vi "laneleftright4.vi"() -> (2 "Coeff right":dbl[](array[numeric]), 3 "Coeff left":dbl[](array[numeric]))   [LabVIEW 2015]
uses:
  G_SEN.vi
  <vilib>/Analysis/1siggen.llb/Ramp Pattern by Delta.vi
  G_LCM.vi
  <vilib>/Analysis/polynomials.llb/1D Polynomial Evaluation (DBL).vi
  G_ALL.vi
  <vilib>/Analysis/NI_AALPro.lvlib
  <vilib>/Analysis/NI_AALBase.lvlib
panel:
  in  "y_gain":dbl min=-1.0 max=1.0
  out "Numeric 2":i32
  out "map_track 2":dbl[][](array[numeric])
  in  "d_safe":dbl=1.0 format="%#_13g"
  out "map_track":dbl[][](array[numeric])
  out "lane_pt":dbl[][](array[numeric])
  in  "x_shift":dbl format="%#_13g"
  in  "y_shift":dbl=-0.0 format="%#_13g"
  in  "x_gain":dbl=0.5 min=-1.0 max=1.0
  out "Lane_C_M":dbl[](array[numeric])=[0.8601491478953653, 0.8717844136967624, 0.882947592858927, 0.8936326403234123, 0.9038337699485205, 0.9135454576426009, 0.9227624443554423, 0.9314797389261423, 0.9396926207859084, 0.9473966425143293, 0.9545876322477319, 0.9612616959383189, 0.9674152194628639, 0.9730448705798238, 0.9781476007338057, 0.9827206467064133, 0.9867615321125792, 0.9902680687415704, 0.993238357741943, 0.9956707906498045, 0.9975640502598242, 0.9989171113385246, 0.9997292411794617, 1.0, 0.9997292411794617, 0.9989171113385246, 0.9975640502598242, 0.9956707906498045, 0.993238357741943, 0.9902680687415704, 0.9867615321125792, 0.9827206467064133]
  out "ratio(-1:left1:right)":dbl
  out "NaN/Path/Refnum?":bool
  out "Rleft":dbl
  out "Rright":dbl
  in  "poly":i32=2 min=1 max=4 step=1
  out "Coeff stop":dbl[](array[numeric])
  out "y_end":dbl[](array[numeric])=[0.8601491478953653, 0.8717844136967624, 0.882947592858927, 0.8936326403234123, 0.9038337699485205, 0.9135454576426009, 0.9227624443554423, 0.9314797389261423, 0.9396926207859084, 0.9473966425143293, 0.9545876322477319, 0.9612616959383189, 0.9674152194628639, 0.9730448705798238, 0.9781476007338057, 0.9827206467064133, 0.9867615321125792, 0.9902680687415704, 0.993238357741943, 0.9956707906498045, 0.9975640502598242, 0.9989171113385246, 0.9997292411794617, 1.0, 0.9997292411794617, 0.9989171113385246, 0.9975640502598242, 0.9956707906498045, 0.993238357741943, 0.9902680687415704, 0.9867615321125792, 0.9827206467064133]
  in  "iter":i32=7
  out "Waveform Graph":dbl[](graph)
  out "w":dbl[](array[numeric])
  out "XY Graph 4":cluster{"Y":dbl[], "Y":dbl[]}[](graph)=[{"Y"=array[3210 elements], "Y"=array[3210 elements]}, {"Y"=[-0.0, 0.001154394197769193, 0.004617650635850623, 0.010389990872226917, 0.018471784248973222, 0.02886354801042046, 0.041565947468740205, 0.056579796217107514, 0.0739060563904701, 0.0935458389742223, 0.11550040416098284, 0.13977116175580306, 0.16635967162997645, 0.19526764422393228, 0.2264969410994837, 0.26004957554195585, 0.2959277132125635, 0.3341336728515216, 0.374669927032528, 0.417539102969144, 0.4627439833735707, 0.5102875073687159, 0.560172771454063, 0.6124030305261954, 0.6669816989546717, 0.7239123517142048, 0.7831987255740245, 0.8448447203451934, 0.9088544001870815, 0.975231994973953, 1.0439819017227023, 1.1151086860829622, 1.1886170838907617, 1.2645120027869723, 1.342798523901962, 1.42348190360768, 1.5065675753387922, 1.592061151484188, 1.6799684253507792, 1.770295373200753, 1.8630481563645134, 1.9582331234307588, 2.0558568125157564, 2.1559259536137603, 2.258447471030621], "Y"=[0.0, 0.5, 1.0, 1.5, 2.0, 2.5, 3.0, 3.5, 4.0, 4.5, 5.0, 5.5, 6.0, 6.5, 7.0, 7.5, 8.0, 8.5, 9.0, 9.5, 10.0, 10.5, 11.0, 11.5, 12.0, 12.5, 13.0, 13.5, 14.0, 14.5, 15.0, 15.5, 16.0, 16.5, 17.0, 17.5, 18.0, 18.5, 19.0, 19.5, 20.0, 20.5, 21.0, 21.5, 22.0]}, {"Y"=[0.362252581831572], "Y"=[-0.8199241909738847]}, {"Y"=array[210 elements], "Y"=array[210 elements]}, {"Y"=[-0.925, -0.925, -0.925, -0.6775, -0.6775, -0.925, -0.925, -0.925, -0.925, -0.6775, -0.6775, -0.925, -0.925, -0.925, 0.9025, 0.9025, 0.9025, 0.6775, 0.6775, 0.9025, 0.9025, 0.9025, 0.9025, 0.6775, 0.6775, 0.9025, 0.9025, 0.9025, -0.925], "Y"=[-0.75, -0.224, 0.224, 0.224, -0.224, -0.224, 0.224, 2.415, 2.885, 2.885, 2.415, 2.415, 2.885, 3.5, 3.5, 2.885, 2.415, 2.415, 2.885, 2.885, 2.415, 0.224, -0.224, -0.224, 0.224, 0.224, -0.224, -0.75, -0.75]}, {"Y"=[0.171875, 0.15377271904051304, 0.1346290179491043, 0.11445423440635205, 0.09325870609283447, 0.07105277068912982, 0.04784676587581635, 0.02365102933347224, -0.0015241012573242174, -0.02766828821599482, -0.05477119386196136, -0.08282248051464558, -0.11181181049346922, -0.14172884611785413, -0.17256324970722198, -0.20430468358099463, -0.23694281005859374, -0.27046729145944115, -0.30486779010295867, -0.340133968308568, -0.3762554883956909, -0.41322201268374914, -0.4510232034921646, -0.4896487231403589], "Y"=[0.0, 0.5, 1.0, 1.5, 2.0, 2.5, 3.0, 3.5, 4.0, 4.5, 5.0, 5.5, 6.0, 6.5, 7.0, 7.5, 8.0, 8.5, 9.0, 9.5, 10.0, 10.5, 11.0, 11.5]}, {"Y"=[1.796875, 1.778772719040513, 1.7596290179491043, 1.739454234406352, 1.7182587060928345, 1.6960527706891297, 1.6728467658758164, 1.6486510293334722, 1.6234758987426758, 1.5973317117840051, 1.5702288061380387, 1.5421775194853544, 1.513188189506531, 1.483271153882146, 1.452436750292778, 1.4206953164190055, 1.3880571899414063, 1.354532708540559, 1.3201322098970414, 1.284866031691432, 1.248744511604309, 1.2117779873162509, 1.1739767965078354, 1.135351276859641, 1.0959117660522462, 1.0556686017662287, 1.014632121682167, 0.9728126634806396, 0.9302205648422242, 0.8868661634474992], "Y"=[0.0, 0.5, 1.0, 1.5, 2.0, 2.5, 3.0, 3.5, 4.0, 4.5, 5.0, 5.5, 6.0, 6.5, 7.0, 7.5, 8.0, 8.5, 9.0, 9.5, 10.0, 10.5, 11.0, 11.5, 12.0, 12.5, 13.0, 13.5, 14.0, 14.5]}, {"Y"=[-1.453125, -1.471227280959487, -1.4903709820508957, -1.510545765593648, -1.5317412939071655, -1.5539472293108703, -1.5771532341241836, -1.6013489706665278, -1.6265241012573242, -1.6526682882159949, -1.6797711938619613, -1.7078224805146456, -1.736811810493469, -1.766728846117854, -1.797563249707222, -1.8293046835809945, -1.8619428100585937, -1.895467291459441, -1.9298677901029586], "Y"=[0.0, 0.5, 1.0, 1.5, 2.0, 2.5, 3.0, 3.5, 4.0, 4.5, 5.0, 5.5, 6.0, 6.5, 7.0, 7.5, 8.0, 8.5, 9.0]}, {"Y"=[0.171875, 0.2568230007600336, 0.3384052130063493, 0.44574342526006827, 0.5205081969556753, 0.5917680690742042, 0.659409530134929, 0.7229937549325056, 0.7835496148685115, 0.8405449546633443, 0.9258576868463875], "Y"=[-20.239964538708662, -19.725637940364884, -19.211158961966362, -18.6998967366845, -18.19022720070031, -17.681887266143153, -17.17615515566314, -16.67683575591291, -16.176265245349786, -15.679082775270938, -15.183754484614711]}, {"Y"=[7.134647485270904], "Y"=[38.71960961082238]}, {"Y"=array[980 elements], "Y"=array[980 elements]}, {"Y"=[], "Y"=[]}]
  out "y":dbl[](array[numeric])
  out "x":dbl[](array[numeric])
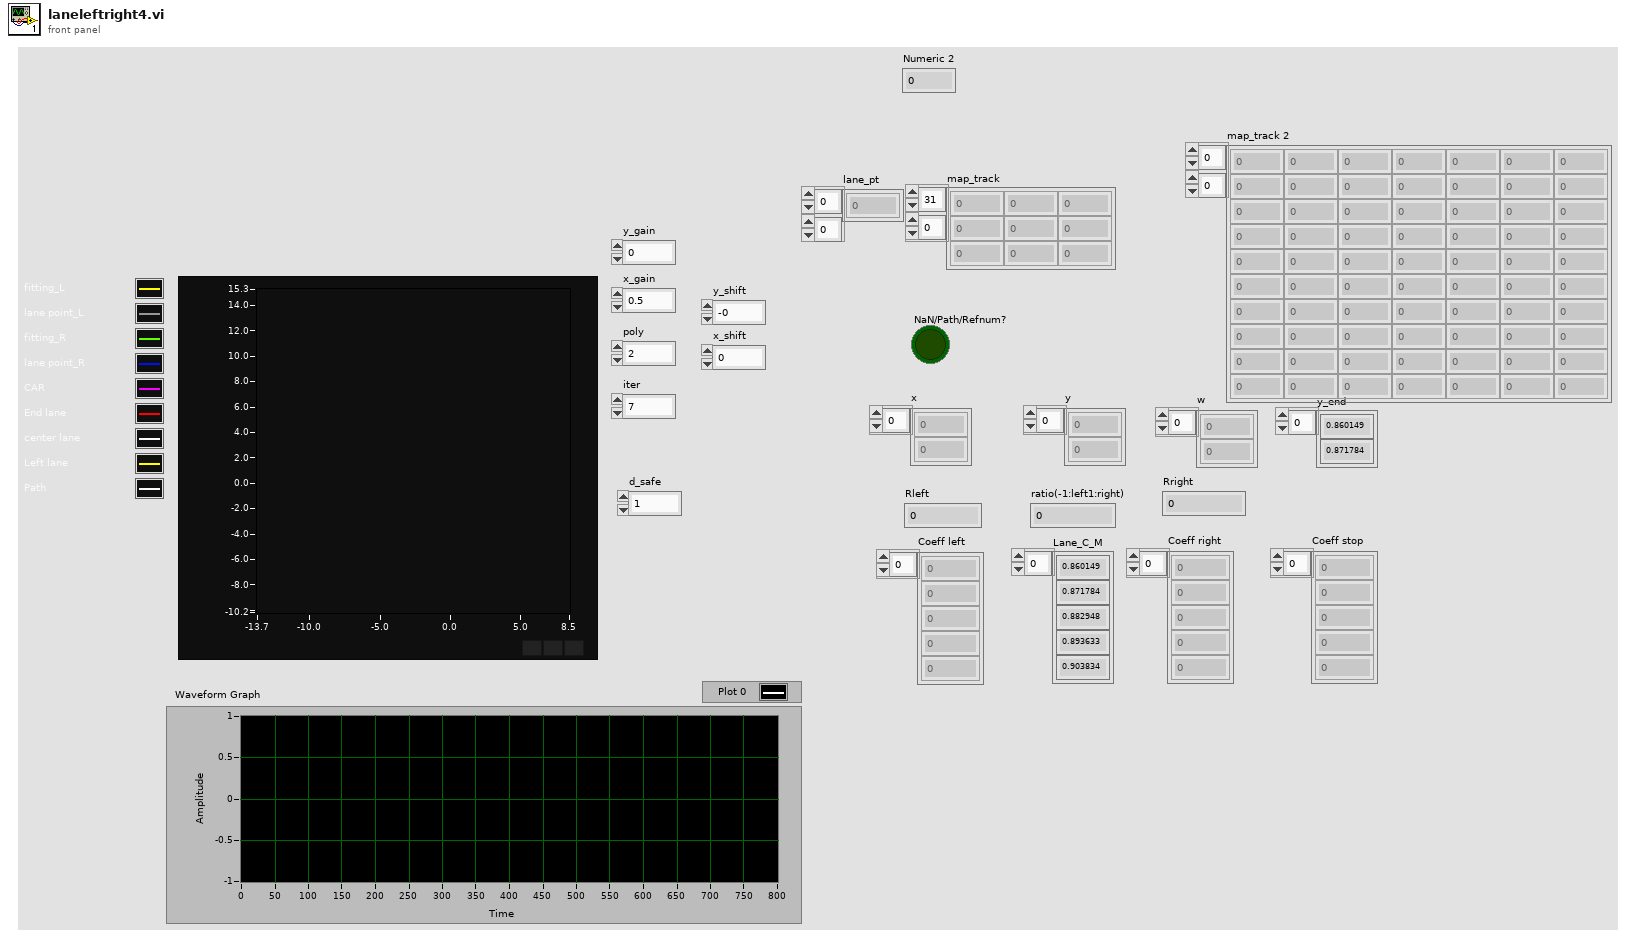
[diagram p1: front panel]
types:
  T1 = cluster{"hash":i64, "sys time":i64, "size":i64, "x":dbl[], "y":dbl[]}
  T2 = cluster{"delta":bool, "Rotational position":dbl, "Rotational position":dbl}[]
  T3 = cluster{"C_Wheel base":dbl, "ratio_steer":dbl, "Overall width":dbl, "af":dbl, "turn radius":dbl, "eval":dbl, "ap":dbl, "an":dbl, "Vmax":dbl, "mu":dbl, "Vlast":dbl}
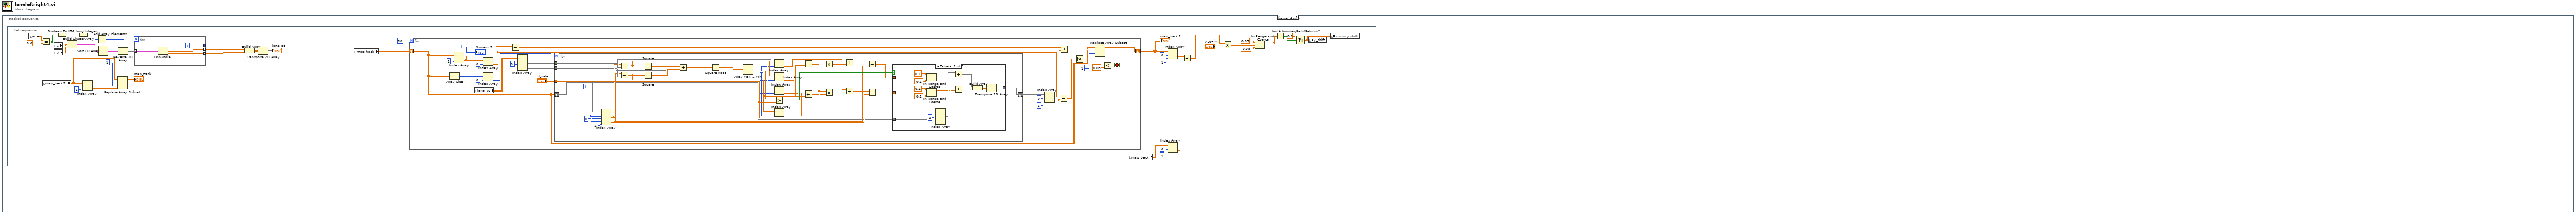
[diagram p0: block diagram]
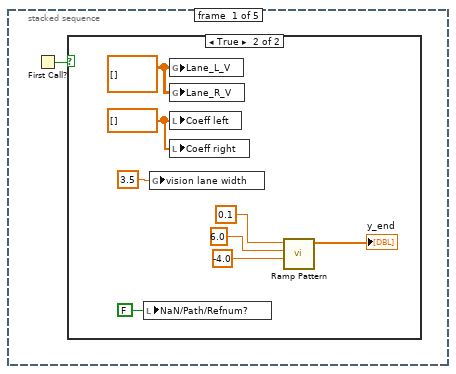
[diagram p2: hidden frame]
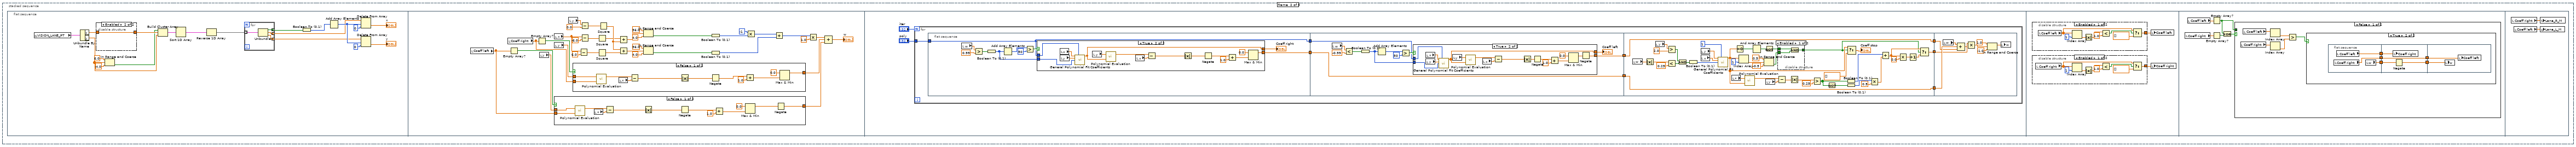
[diagram p4: hidden frame]
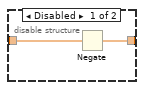
[diagram p5: hidden frame]
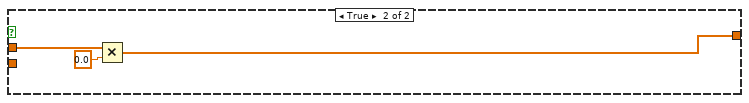
[diagram p6: hidden frame]
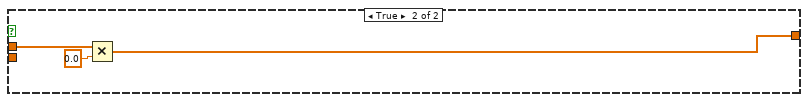
[diagram p7: hidden frame]
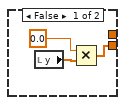
[diagram p8: hidden frame]
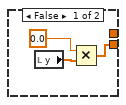
[diagram p9: hidden frame]
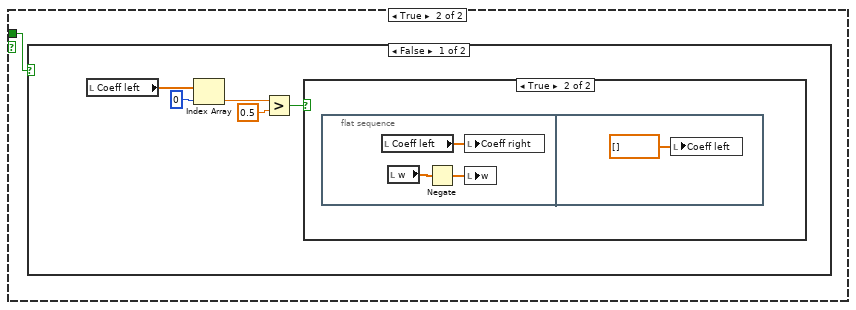
[diagram p14: hidden frame]
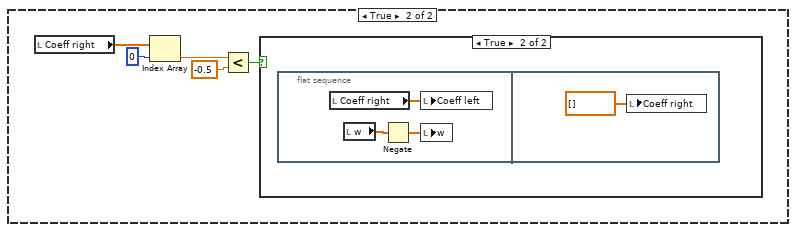
[diagram p16: hidden frame]
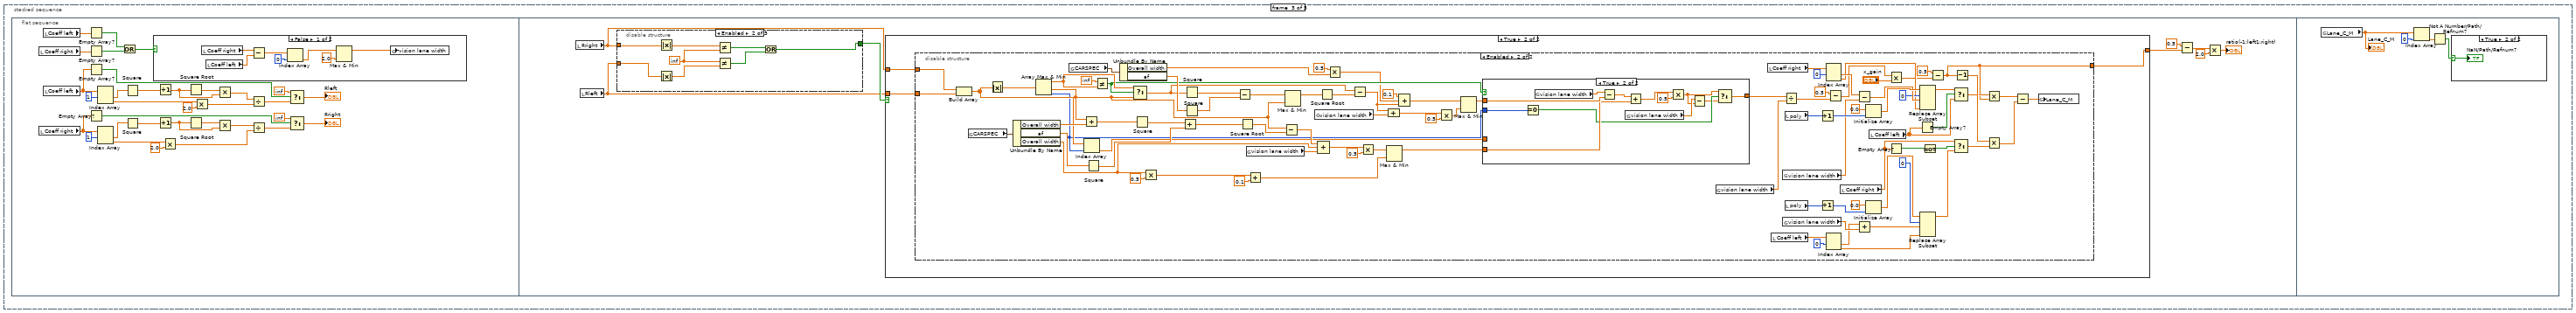
[diagram p18: hidden frame]
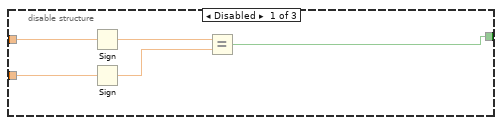
[diagram p20: hidden frame]
diagram:
  n1 = stacked-sequence {
    frame #0 {
      n2 = First Call?() -> (First Call?: T/F=w1:bool)
      n3 = case shown="True" w1 {
        frame False {
        }
        frame True {
          w2 = dbl[] [] ("Coeff left")
          w4 = dbl[][] [] ("Lane_R_V")
          n4 = local write "NaN/Path/Refnum?"(FALSE ("NaN/Path/Refnum?")) -> ()
          n5 = global write "G_SEN.vi" "vision lane width"(3.5 ("vision lane width")) -> ()
          n6 = global write "G_SEN.vi" "Lane_L_V"(w4) -> ()
          n7 = global write "G_SEN.vi" "Lane_R_V"(w4) -> ()
          n8 = local write "Coeff left"(w2) -> ()
          n9 = local write "Coeff right"(w2) -> ()
          n10 = call-poly <vilib>:"Ramp Pattern.vi"("start"=-4.0, "end"=6.0, "delta"=0.1) -> ("Ramp Pattern"=→"y_end":dbl[])  [unwired: 6 in, 2 out]
        }
      }
    }
    frame #1 {
      n11 = flat-sequence {
        frame #0 {
          n12 = global read "G_LCM.vi" "VISION_LANE_PT"() -> (w10:T1)
          n13 = Unbundle By Name(w10) -> ("x"=w27:dbl[], "y"=w21:dbl[])
          n14 = disable-structure shown="Enabled" {
            disable-tunnel: w27 -> [w30 w31]
            disable-tunnel: [w29 w31] -> w28
            frame Disabled {
              n15 = Negate(x=w30) -> (-x=w29:dbl[])
            }
            frame Enabled {
            }
          }
          n16 = In Range and Coerce(upper limit=6.0 ("delta"), x=w21, lower limit=-4.0) -> (In Range?=w19:bool[])  [unwired: 1 out]
          n17 = Build Cluster Array(w19, w28, w21) -> (w17:T2)
          n18 = Sort 1D Array(array=w17) -> (sorted array=w18:T2)
          n19 = Reverse 1D Array(array=w18) -> (reversed array=w12:T2)
          n20 = for {
            tunnel: w12 -> [w35] mode=indexing
            tunnel: [w34] -> w14 mode=indexing
            tunnel: [w33] -> w15 mode=indexing
            tunnel: [w32] -> w22 mode=indexing
            n21 = Unbundle(w35) -> ("delta"=w32:bool, "Rotational position"=w34:dbl, "Rotational position"=w33:dbl)
          }
          n22 = Boolean To (0,1)(Boolean=w22) -> (0, 1=w13:i16[])
          n23 = Add Array Elements(numeric array=w13) -> (sum=w23:i16)
          n24 = Delete From Array(array=w14, length=w23, index=0) -> (deleted portion=→"x":dbl[])  [unwired: 1 out]
          n25 = Delete From Array(array=w15, length=w23, index=0) -> (deleted portion=→"y":dbl[])  [unwired: 1 out]
        }
        frame #1 {
          n26 = local read "Coeff left"() -> (w67:dbl[])
          n27 = local read "Coeff right"() -> (w66:dbl[])
          n28 = Empty Array?(array=w67) -> (empty?=w68:bool)
          n29 = Empty Array?(array=w66) -> (empty?=w69:bool)
          n30 = local read "y"() -> (w64:dbl[])
          n31 = local read "x"() -> (w36:dbl[])
          n32 = local read "y"() -> (w70:dbl[])
          n33 = case shown="False" w68 {
            tunnel: w64 -> [w90 w98]
            tunnel: w67 -> [w87 _]
            tunnel: [w85 w97] -> w65
            frame False {
              n34 = call-poly <vilib>:"Polynomial Evaluation.vi"("P(x)"=w87, "A"=w90) -> ("P(A)"=w89:dbl[])  [unwired: 1 out]
              n35 = local read "x"() -> (w88:dbl[])
              n36 = Subtract(x=w89, y=w88) -> (x-y=w94:dbl[])
              n37 = Absolute Value(x=w94) -> (abs(x)=w93:dbl[])
              n38 = Negate(x=w93) -> (-x=w92:dbl[])
              n39 = Add(x=w92, y=1.0) -> (x+y=w96:dbl[])
              n40 = Max & Min(x=0.0, y=w96) -> (max(x,y)=w86:dbl[])  [unwired: 1 out]
              n41 = Negate(x=w86) -> (-x=w85:dbl[])
            }
            frame True {
              n42 = Multiply(x=w98, y=0.0) -> (x*y=w97:dbl[])
            }
          }
          n43 = local read "y"() -> (w37:dbl[])
          n44 = case shown="False" w69 {
            tunnel: [w79 w82] -> w62
            tunnel: w66 -> [w78 _]
            tunnel: w70 -> [w71 w83]
            frame False {
              n45 = call-poly <vilib>:"Polynomial Evaluation.vi"("P(x)"=w78, "A"=w71) -> ("P(A)"=w76:dbl[])  [unwired: 1 out]
              n46 = local read "x"() -> (w77:dbl[])
              n47 = Subtract(x=w76, y=w77) -> (x-y=w72:dbl[])
              n48 = Absolute Value(x=w72) -> (abs(x)=w73:dbl[])
              n49 = Negate(x=w73) -> (-x=w74:dbl[])
              n50 = Add(x=w74, y=1.0) -> (x+y=w80:dbl[])
              n51 = Max & Min(x=0.0, y=w80) -> (max(x,y)=w79:dbl[])  [unwired: 1 out]
            }
            frame True {
              n52 = Multiply(x=w83, y=0.0) -> (x*y=w82:dbl[])
            }
          }
          n53 = Subtract(x=w36, y=6.0) -> (x-y=w40:dbl[])
          n54 = Subtract(x=w37, y=0.0) -> (x-y=w49:dbl[])
          n55 = Subtract(x=w36, y=-6.0) -> (x-y=w42:dbl[])
          n56 = Square(x=w42) -> (x^2=w41:dbl[])
          n57 = Square(x=w40) -> (x^2=w50:dbl[])
          n58 = Square(x=w49) -> (x^2=w51:dbl[])
          n59 = Add(x=w41, y=w51) -> (x+y=w57:dbl[])
          n60 = Add(x=w51, y=w50) -> (x+y=w52:dbl[])
          n61 = In Range and Coerce(upper limit=36.0, x=w57, lower limit=4.0) -> (In Range?=w59:bool[])  [unwired: 1 out]
          n62 = In Range and Coerce(upper limit=36.0, x=w52, lower limit=4.0) -> (In Range?=w58:bool[])  [unwired: 1 out]
          n63 = Boolean To (0,1)(Boolean=w59) -> (0, 1=w60:i16[])
          n64 = Boolean To (0,1)(Boolean=w58) -> (0, 1=w61:i16[])
          n65 = Multiply(x=i16 -1, y=w60) -> (x*y=w45:i16[])
          n66 = Add(x=w45, y=w61) -> (x+y=w47:i16[])
          n67 = Multiply(x=w47, y=1.0 ("element")) -> (x*y=w63:dbl[])
          n68 = Compound Arithmetic op=ADD(w63, w62, w65) -> (→"w":dbl[])
        }
        frame #2 {
          n69 = for {
            N: "iter" -> [_]
            tunnel: "poly" -> [w103]
            n70 = flat-sequence {
              tunnel: [w117] -> w109
              tunnel: w103 -> [w110]
              tunnel: [w110] -> w102
              tunnel: [w148] -> w108
              tunnel: w109 -> [w148]
              tunnel: [w145] -> w106
              tunnel: w102 -> [w138]
              tunnel: w108 -> [w210]
              tunnel: [w210] -> w107
              tunnel: w106 -> [w209]
              tunnel: [w209] -> w105
              tunnel: [w180] -> w104
              tunnel: w107 -> [w218]
              tunnel: w105 -> [w217]
              tunnel: w104 -> [w216]
              frame #0 {
                n71 = local read "w"() -> (w119:dbl[])
                n72 = Greater?(x=w119, y=0.99) -> (0:w111:bool[])
                n73 = Boolean To (0,1)(Boolean=w111) -> (0, 1=w112:i16[])
                n74 = Add Array Elements(numeric array=w112) -> (sum=w115:i16)
                n75 = Greater?(x=w115, y=i16 50) -> (0:w113:bool)
                n76 = case shown="True" w113 {
                  tunnel: [w121 w128] -> w117
                  tunnel: [_ w127] -> w116
                  tunnel: w112 -> [_ w124]
                  tunnel: w110 -> [_ w123]
                  frame False {
                    n77 = local read "y"() -> (w122:dbl[])
                    n78 = Multiply(x=0.0, y=w122) -> (x*y=w121:dbl[])
                  }
                  frame True {
                    n79 = local read "x"() -> (w125:dbl[])
                    n80 = local read "y"() -> (w126:dbl[])
                    n81 = call <vilib>:"General Polynomial Fit Coefficients.vi"("Y"=w125, "polynomial order"=w123, "X"=w126, "Weight"=w124) -> ("Polynomial Coefficients"=w127:dbl[])  [unwired: 10 in, 1 out]
                    n82 = local read "y"() -> (w137:dbl[])
                    n83 = call-poly <vilib>:"Polynomial Evaluation.vi"("P(x)"=w127, "A"=w137) -> ("P(A)"=w136:dbl[])  [unwired: 1 out]
                    n84 = local read "x"() -> (w135:dbl[])
                    n85 = Subtract(x=w136, y=w135) -> (x-y=w134:dbl[])
                    n86 = Absolute Value(x=w134) -> (abs(x)=w133:dbl[])
                    n87 = Negate(x=w133) -> (-x=w132:dbl[])
                    n88 = Add(x=w132, y=1.0) -> (x+y=w129:dbl[])
                    n89 = Max & Min(x=0.0, y=w129) -> (max(x,y)=w128:dbl[])  [unwired: 1 out]
                  }
                }
                "Coeff right" <- w116
              }
              frame #1 {
                n90 = local read "w"() -> (w146:dbl[])
                n91 = Less?(x=w146, y=-0.99) -> (x < y?=w141:bool[])
                n92 = Boolean To (0,1)(Boolean=w141) -> (0, 1=w139:i16[])
                n93 = Add Array Elements(numeric array=w139) -> (sum=w142:i16)
                n94 = Greater?(x=w142, y=i16 50) -> (0:w140:bool)
                n95 = case shown="True" w140 {
                  tunnel: [w149 w157] -> w145
                  tunnel: [_ w156] -> w144
                  tunnel: w139 -> [_ w153]
                  tunnel: w138 -> [_ w152]
                  frame False {
                    n96 = local read "y"() -> (w150:dbl[])
                    n97 = Multiply(x=0.0, y=w150) -> (x*y=w149:dbl[])
                  }
                  frame True {
                    n98 = local read "x"() -> (w154:dbl[])
                    n99 = local read "y"() -> (w155:dbl[])
                    n100 = call <vilib>:"General Polynomial Fit Coefficients.vi"("Y"=w154, "polynomial order"=w152, "X"=w155, "Weight"=w153) -> ("Polynomial Coefficients"=w156:dbl[])  [unwired: 10 in, 1 out]
                    n101 = local read "y"() -> (w161:dbl[])
                    n102 = call-poly <vilib>:"Polynomial Evaluation.vi"("P(x)"=w156, "A"=w161) -> ("P(A)"=w162:dbl[])  [unwired: 1 out]
                    n103 = local read "x"() -> (w163:dbl[])
                    n104 = Subtract(x=w162, y=w163) -> (x-y=w164:dbl[])
                    n105 = Absolute Value(x=w164) -> (abs(x)=w165:dbl[])
                    n106 = Negate(x=w165) -> (-x=w159:dbl[])
                    n107 = Add(x=w159, y=1.0) -> (x+y=w166:dbl[])
                    n108 = Max & Min(x=0.0, y=w166) -> (max(x,y)=w160:dbl[])  [unwired: 1 out]
                    n109 = Negate(x=w160) -> (-x=w157:dbl[])
                  }
                }
                "Coeff left" <- w144
              }
              frame #2 {
                n110 = local read "w"() -> (w188:dbl[])
                n111 = Absolute Value(x=w188) -> (abs(x)=w187:dbl[])
                n112 = local read "y"() -> (w192:dbl[])
                n113 = Greater?(x=w192, y=2.0) -> (0:w190:bool[])
                n114 = Less?(x=w187, y=0.25) -> (x < y?=w186:bool[])
                n115 = And(x=w190, y=w186) -> (x .and. y?=w189:bool[])
                n116 = Boolean To (0,1)(Boolean=w189) -> (0, 1=w208:i16[])
                n117 = local read "y"() -> (w202:dbl[])
                n118 = local read "x"() -> (w201:dbl[])
                n119 = call <vilib>:"General Polynomial Fit Coefficients.vi"("Y"=w202, "polynomial order"=1, "X"=w201, "Weight"=w208) -> ("Polynomial Coefficients"=w173:dbl[])  [unwired: 10 in, 1 out]
                n120 = local read "x"() -> (w206:dbl[])
                n121 = Equal To 0?(x=w173) -> (x = 0?=w172:bool[])
                n122 = Index Array(array=w173, index=1) -> (element=w183:dbl)
                n123 = call-poly <vilib>:"Polynomial Evaluation.vi"("P(x)"=w173, "A"=w206) -> ("P(A)"=w205:dbl[])  [unwired: 1 out]
                n124 = And Array Elements(Boolean array=w172) -> (logical AND=w169:bool)
                n125 = In Range and Coerce(upper limit=0.5, x=w183, lower limit=-0.5) -> (In Range?=w171:bool)  [unwired: 1 out]
                n126 = Not(x=w169) -> (.not. x?=w168:bool)
                n127 = local read "y"() -> (w204:dbl[])
                n128 = Subtract(x=w205, y=w204) -> (x-y=w203:dbl[])
                n129 = disable-structure shown="Enabled" {
                  disable-tunnel: w171 -> [w213 _]
                  disable-tunnel: [w212 _] -> w170
                  disable-tunnel: w168 -> [w211 _]
                  frame Enabled {
                    n130 = And(x=w211, y=w213) -> (x .and. y?=w212:bool)
                  }
                  frame Disabled {
                  }
                }
                n131 = Absolute Value(x=w203) -> (abs(x)=w200:dbl[])
                n132 = Greater?(x=w200, y=0.25 ("Numeric 2")) -> (0:w198:bool[])
                n133 = Not(x=w198) -> (.not. x?=w197:bool[])
                n134 = Boolean To (0,1)(Boolean=w198) -> (0, 1=w193:i16[])
                n135 = Boolean To (0,1)(Boolean=w197) -> (0, 1=w196:i16[])
                n136 = Select(t=w173, s=w170, f=dbl[] []) -> (s? t:f=→"Coeff stop":dbl[])
                n137 = Multiply(x=w196, y=0.5) -> (x*y=w194:dbl[])
                n138 = Add(x=w193, y=w194) -> (x+y=w179:dbl[])
                n139 = Multiply(x=w179, y=0.0) -> (x*y=w177:dbl[])
                n140 = Increment(x=w177) -> (x+1=w176:dbl[])
                n141 = Select(t=w179, s=w170, f=w176) -> (s? t:f=w180:dbl[])
              }
              frame #3 {
                n142 = local read "w"() -> (w222:dbl[])
                n143 = Compound Arithmetic op=ADD(w222, w218, w217) -> (w215:dbl[])
                n144 = Multiply(x=w216, y=w215) -> (x*y=w214:dbl[])
                n145 = In Range and Coerce(upper limit=1.0, x=w214, lower limit=-1.0) -> (coerced(x)=w219:dbl[])  [unwired: 1 out]
                n146 = local write "w"(w219) -> ()
              }
            }
          }
        }
        frame #3 {
          n147 = disable-structure shown="Enabled" {
            disable-tunnel: [w226 _] -> w223
            frame Enabled {
              n148 = local read "Coeff left"() -> (w225:dbl[])
              n149 = Index Array(array=w225, index=1) -> (element=w228:dbl)
              n150 = Absolute Value(x=w228) -> (abs(x)=w229:dbl)
              n151 = Less?(x=w229, y=1.0) -> (x < y?=w231:bool)
              n152 = Select(t=w225, s=w231, f=dbl[] []) -> (s? t:f=w226:dbl[])
            }
            frame Disabled {
            }
          }
          n153 = disable-structure shown="Enabled" {
            disable-tunnel: [w235 _] -> w224
            frame Enabled {
              n154 = local read "Coeff right"() -> (w233:dbl[])
              n155 = Index Array(array=w233, index=1) -> (element=w239:dbl)
              n156 = Absolute Value(x=w239) -> (abs(x)=w238:dbl)
              n157 = Less?(x=w238, y=1.0) -> (x < y?=w236:bool)
              n158 = Select(t=w233, s=w236, f=dbl[] []) -> (s? t:f=w235:dbl[])
            }
            frame Disabled {
            }
          }
          n159 = local write "Coeff left"(w223) -> ()
          n160 = local write "Coeff right"(w224) -> ()
        }
        frame #4 {
          n161 = local read "Coeff right"() -> (w242:dbl[])
          n162 = local read "Coeff left"() -> (w241:dbl[])
          n163 = Empty Array?(array=w241) -> (empty?=w245:bool)
          n164 = Empty Array?(array=w242) -> (empty?=w243:bool)
          n165 = Exclusive Or(1:w243, 2:w245) -> (0:w244:bool)
          n166 = case shown="False" w244 {
            tunnel: w245 -> [_ w265]
            frame False {
              n167 = local read "Coeff right"() -> (w249:dbl[])
              n168 = local read "Coeff left"() -> (w250:dbl[])
              n169 = Index Array(array=w250) -> (element=w248:dbl)  [unwired: 1 in]
              n170 = Index Array(array=w249) -> (element=w247:dbl)  [unwired: 1 in]
              n171 = Greater?(x=w248, y=w247) -> (0:w246:bool)
              n172 = case shown="True" w246 {
                frame False {
                }
                frame True {
                  n173 = flat-sequence {
                    tunnel: [w258] -> w254
                    tunnel: [w257] -> w253
                    tunnel: [w256] -> w252
                    tunnel: [w262] -> w255
                    tunnel: w254 -> [w262]
                    tunnel: w253 -> [w261]
                    tunnel: w252 -> [w260]
                    tunnel: [w259] -> w251
                    tunnel: w255 -> [w264]
                    tunnel: w251 -> [w263]
                    frame #0 {
                      n174 = local read "Coeff right"() -> (w258:dbl[])
                      n175 = local read "Coeff left"() -> (w257:dbl[])
                      n176 = local read "w"() -> (w256:dbl[])
                    }
                    frame #1 {
                      n177 = local write "Coeff right"(w261) -> ()
                      n178 = Negate(x=w260) -> (-x=w259:dbl[])
                    }
                    frame #2 {
                      n179 = local write "w"(w263) -> ()
                      n180 = local write "Coeff left"(w264) -> ()
                    }
                  }
                }
              }
            }
            frame True {
              n181 = case shown="False" w265 {
                frame False {
                  n182 = local read "Coeff left"() -> (w270:dbl[])
                  n183 = Index Array(array=w270, index=0) -> (element=w268:dbl)
                  n184 = Greater?(x=w268, y=0.5) -> (0:w266:bool)
                  n185 = case shown="True" w266 {
                    frame False {
                    }
                    frame True {
                      n186 = flat-sequence {
                        frame #0 {
                          n187 = local read "Coeff left"() -> (w273:dbl[])
                          n188 = local read "w"() -> (w272:dbl[])
                          n189 = Negate(x=w272) -> (-x=w271:dbl[])
                          n190 = local write "Coeff right"(w273) -> ()
                          n191 = local write "w"(w271) -> ()
                        }
                        frame #1 {
                          n192 = local write "Coeff left"(dbl[] []) -> ()
                        }
                      }
                    }
                  }
                }
                frame True {
                  n193 = local read "Coeff right"() -> (w279:dbl[])
                  n194 = Index Array(array=w279, index=0) -> (element=w277:dbl)
                  n195 = Less?(x=w277, y=-0.5) -> (x < y?=w275:bool)
                  n196 = case shown="True" w275 {
                    frame False {
                    }
                    frame True {
                      n197 = flat-sequence {
                        frame #0 {
                          n198 = local read "Coeff right"() -> (w282:dbl[])
                          n199 = local read "w"() -> (w281:dbl[])
                          n200 = Negate(x=w281) -> (-x=w280:dbl[])
                          n201 = local write "Coeff left"(w282) -> ()
                          n202 = local write "w"(w280) -> ()
                        }
                        frame #1 {
                          n203 = local write "Coeff right"(dbl[] []) -> ()
                        }
                      }
                    }
                  }
                }
              }
            }
          }
        }
        frame #5 {
          n204 = local read "Coeff right"() -> (w285:dbl[])
          n205 = local read "Coeff left"() -> (w284:dbl[])
          n206 = global write "G_SEN.vi" "Lane_R_M"(w285) -> ()
          n207 = global write "G_SEN.vi" "Lane_L_M"(w284) -> ()
        }
      }
    }
    frame #2 {
      n208 = flat-sequence {
        frame #0 {
          n209 = local read "Coeff right"() -> (w287:dbl[])
          n210 = local read "Coeff right"() -> (w315:dbl[])
          n211 = local read "Coeff left"() -> (w286:dbl[])
          n212 = local read "Coeff left"() -> (w313:dbl[])
          n213 = Empty Array?(array=w286) -> (empty?=w289:bool)
          n214 = Empty Array?(array=w287) -> (empty?=w290:bool)
          n215 = Empty Array?(array=w313) -> (empty?=w307:bool)
          n216 = Empty Array?(array=w315) -> (empty?=w309:bool)
          n217 = Index Array(array=w313, index #1=1 ("index")) -> (element #1=w306:dbl, element #2=w299:dbl)  [unwired: 1 in]
          n218 = Index Array(array=w315, index #1=1 ("index")) -> (element #1=w291:dbl, element #2=w298:dbl)  [unwired: 1 in]
          n219 = Or(x=w289, y=w290) -> (x .or. y?=w288:bool)
          n220 = Square(x=w306) -> (x^2=w305:dbl)
          n221 = Square(x=w291) -> (x^2=w292:dbl)
          n222 = case shown="False" w288 {
            frame False {
              n223 = local read "Coeff right"() -> (w322:dbl[])
              n224 = local read "Coeff left"() -> (w319:dbl[])
              n225 = Subtract(x=w322, y=w319) -> (x-y=w320:dbl[])
              n226 = Index Array(array=w320, index=0) -> (element=w323:dbl)
              n227 = Max & Min(x=w323, y=2.0) -> (max(x,y)=w324:dbl)  [unwired: 1 out]
              n228 = global write "G_SEN.vi" "vision lane width"(w324) -> ()
            }
            frame True {
            }
          }
          n229 = Increment(x=w305) -> (x+1=w303:dbl)
          n230 = Increment(x=w292) -> (x+1=w294:dbl)
          n231 = Multiply(x=w298, y=2.0) -> (x*y=w296:dbl)
          n232 = Square Root(x=w303) -> (sqrt(x)=w304:dbl)
          n233 = Square Root(x=w294) -> (sqrt(x)=w293:dbl)
          n234 = Multiply(x=w299, y=2.0) -> (x*y=w301:dbl)
          n235 = Multiply(x=w304, y=w303) -> (x*y=w302:dbl)
          n236 = Multiply(x=w293, y=w294) -> (x*y=w295:dbl)
          n237 = Divide(x=w302, y=w301) -> (x/y=w308:dbl)
          n238 = Divide(x=w295, y=w296) -> (x/y=w310:dbl)
          n239 = Select(t=inf, s=w307, f=w308) -> (s? t:f=→"Rleft":dbl)
          n240 = Select(t=inf, s=w309, f=w310) -> (s? t:f=→"Rright":dbl)
        }
        frame #1 {
          n241 = local read "Rright"() -> (w326:dbl)
          n242 = local read "Rleft"() -> (w327:dbl)
          n243 = disable-structure shown="Enabled" {
            disable-tunnel: w326 -> [w338 w345 _]
            disable-tunnel: w327 -> [w337 w346 _]
            disable-tunnel: [w334 w341 TRUE] -> w328
            frame Disabled {
              n244 = Sign(1:w338) -> (0:w336:dbl)
              n245 = Sign(1:w337) -> (0:w335:dbl)
              n246 = Equal?(x=w336, y=w335) -> (x = y?=w334:bool)
            }
            frame Enabled {
              w343 = inf
              n247 = Absolute Value(x=w345) -> (abs(x)=w344:dbl)
              n248 = Absolute Value(x=w346) -> (abs(x)=w342:dbl)
              n249 = Not Equal?(x=w344, y=w343) -> (x != y?=w340:bool)
              n250 = Not Equal?(x=w343, y=w342) -> (x != y?=w339:bool)
              n251 = Or(x=w340, y=w339) -> (x .or. y?=w341:bool)
            }
            frame Disabled {
            }
          }
          n252 = case shown="True" w328 {
            tunnel: w326 -> [_ w383]
            tunnel: w327 -> [_ w382]
            tunnel: [0.5 w381] -> w329
            frame False {
              n253 = local read "Coeff right"() -> (w352:dbl[])
              n254 = local read "Coeff left"() -> (w353:dbl[])
              n255 = Empty Array?(array=w352) -> (empty?=w351:bool)
              n256 = Empty Array?(array=w353) -> (empty?=w349:bool)
              n257 = Exclusive Or(1:w351, 2:w349) -> (0:w350:bool)
              n258 = case shown="True" w350 {
                tunnel: w349 -> [w354 w362]
                frame False {
                  n259 = case shown="True" w354 {
                    frame False {
                      w355 = 0.5
                      n260 = local read "Coeff right"() -> (w359:dbl[])
                      n261 = local read "Coeff left"() -> (w361:dbl[])
                      n262 = Decrement(x=w355) -> (x-1=w360:dbl)
                      n263 = Multiply(x=w361, y=w355) -> (x*y=w358:dbl[])
                      n264 = Multiply(x=w360, y=w359) -> (x*y=w357:dbl[])
                      n265 = Subtract(x=w358, y=w357) -> (x-y=w356:dbl[])
                      n266 = global write "G_SEN.vi" "Lane_C_M"(w356) -> ()
                    }
                    frame True {
                    }
                  }
                }
                frame True {
                  n267 = case shown="False" w362 {
                    frame False {
                      n268 = global read "G_SEN.vi" "vision lane width"() -> (w365:dbl)
                      n269 = local read "Coeff left"() -> (w371:dbl[])
                      n270 = Index Array(array=w371, index=0) -> (element=w369:dbl)
                      n271 = Multiply(x=w365, y=0.5) -> (x*y=w363:dbl)
                      n272 = Add(x=w369, y=w363) -> (x+y=w368:dbl)
                      n273 = Replace Array Subset(array=w371, new element=w368, index=0) -> (w366:dbl[])
                      n274 = global write "G_SEN.vi" "Lane_C_M"(w366) -> ()
                    }
                    frame True {
                      n275 = global read "G_SEN.vi" "vision lane width"() -> (w374:dbl)
                      n276 = local read "Coeff right"() -> (w380:dbl[])
                      n277 = Index Array(array=w380, index=0) -> (element=w378:dbl)
                      n278 = Multiply(x=w374, y=0.5) -> (x*y=w372:dbl)
                      n279 = Subtract(x=w378, y=w372) -> (x-y=w377:dbl)
                      n280 = Replace Array Subset(array=w380, new element=w377, index=0) -> (w375:dbl[])
                      n281 = global write "G_SEN.vi" "Lane_C_M"(w375) -> ()
                    }
                  }
                }
              }
            }
            frame True {
              n282 = disable-structure shown="Enabled" {
                disable-tunnel: w383 -> [w392 w616]
                disable-tunnel: w382 -> [w391 w615]
                disable-tunnel: [_ w543] -> w381
                frame Disabled {
                  n283 = Absolute Value(x=w392) -> (abs(x)=w414:dbl)
                  n284 = Absolute Value(x=w391) -> (abs(x)=w413:dbl)
                  n285 = global read "G_ALL.vi" "CARSPEC"() -> (w409:T3)
                  n286 = global read "G_ALL.vi" "CARSPEC"() -> (w430:T3)
                  n287 = Build Array(w414, w413) -> (w412:dbl[])
                  n288 = Unbundle By Name(w409) -> ("af"=w408:dbl, "Overall width"=w398:dbl)
                  n289 = Unbundle By Name(w430) -> ("Overall width"=w419:dbl, "af"=w427:dbl, "Overall width"=w415:dbl)
                  n290 = Array Max & Min(array=w412) -> (min value=w405:dbl, min index (indices)=w411:i32)  [unwired: 2 out]
                  n291 = Add(x=w405, y=w419) -> (x+y=w429:dbl)
                  n292 = Square(x=w405) -> (x^2=w396:dbl)
                  n293 = Square(x=w408) -> (x^2=w395:dbl)
                  n294 = Multiply(x=w398, y=0.5) -> (x*y=w397:dbl)
                  n295 = Square(x=w429) -> (x^2=w428:dbl)
                  n296 = Square(x=w427) -> (x^2=w420:dbl)
                  n297 = Subtract(x=w396, y=w395) -> (x-y=w390:dbl)
                  n298 = Multiply(x=w415, y=0.5) -> (x*y=w416:dbl)
                  n299 = Add(x=w428, y=w420) -> (x+y=w426:dbl)
                  n300 = Square Root(x=w390) -> (sqrt(x)=w407:dbl)
                  n301 = Subtract(x=w407, y=w398) -> (x-y=w406:dbl)
                  n302 = Square Root(x=w426) -> (sqrt(x)=w424:dbl)
                  n303 = global read "G_SEN.vi" "vision lane width"() -> (w401:dbl)
                  n304 = global read "G_SEN.vi" "vision lane width"() -> (w425:dbl)
                  n305 = Subtract(x=w405, y=w406) -> (x-y=w400:dbl)
                  n306 = Subtract(x=w424, y=w405) -> (x-y=w423:dbl)
                  n307 = Subtract(x=w401, y=w400) -> (x-y=w402:dbl)
                  n308 = Subtract(x=w425, y=w423) -> (x-y=w422:dbl)
                  n309 = global read "G_SEN.vi" "vision lane width"() -> (w386:dbl)
                  n310 = global read "G_SEN.vi" "vision lane width"() -> (w393:dbl)
                  n311 = Multiply(x=w402, y=0.5) -> (x*y=w404:dbl)
                  n312 = Multiply(x=w422, y=0.5) -> (x*y=w417:dbl)
                  n313 = Compound Arithmetic op=ADD(w404, w397) -> (w394:dbl)
                  n314 = Compound Arithmetic op=ADD(w417, w416) -> (w410:dbl)
                  n315 = Subtract(x=w393, y=w394) -> (x-y=w388:dbl)
                  n316 = Less Than 0?(x=w390) -> (x < 0?=w389:bool)
                  n317 = Multiply(x=0.5 ("y"), y=w386) -> (x*y=w385:dbl)
                  n318 = Select(t=w385, s=w389, f=w388) -> (s? t:f=w387:dbl)
                  n319 = case shown="1" w411 {
                    tunnel: w410 -> [w432 w480]
                    tunnel: w387 -> [w431 w478]
                    frame 0, Default {
                      n320 = local read "Rright"() -> (w434:dbl)
                      n321 = Greater Than 0?(x=w434) -> (x > 0?=w433:bool)
                      n322 = case shown="True" w433 {
                        tunnel: w432 -> [_ w455]
                        tunnel: w431 -> [w437 w454]
                        frame False {
                          n323 = local read "Coeff left"() -> (w436:dbl[])
                          n324 = Empty Array?(array=w436) -> (empty?=w435:bool)
                          n325 = case shown="False" w435 {
                            tunnel: w437 -> [w438 w447]
                            frame False {
                              n326 = global read "G_SEN.vi" "vision lane width"() -> (w446:dbl)
                              n327 = Divide(x=w438, y=w446) -> (x/y=w444:dbl)
                              n328 = local read "Coeff right"() -> (w442:dbl[])
                              n329 = local read "Coeff left"() -> (w445:dbl[])
                              n330 = Decrement(x=w444) -> (x-1=w443:dbl)
                              n331 = Multiply(x=w445, y=w444) -> (x*y=w441:dbl[])
                              n332 = Multiply(x=w443, y=w442) -> (x*y=w440:dbl[])
                              n333 = Subtract(x=w441, y=w440) -> (x-y=w439:dbl[])
                              n334 = global write "G_SEN.vi" "Lane_C_M"(w439) -> ()
                            }
                            frame True {
                              n335 = local read "Coeff right"() -> (w453:dbl[])
                              n336 = Index Array(array=w453, index=0) -> (element=w451:dbl)
                              n337 = Subtract(x=w451, y=w447) -> (x-y=w450:dbl)
                              n338 = Replace Array Subset(array=w453, new element=w450, index=0) -> (w448:dbl[])
                              n339 = global write "G_SEN.vi" "Lane_C_M"(w448) -> ()
                            }
                          }
                        }
                        frame True {
                          n340 = local read "Coeff left"() -> (w457:dbl[])
                          n341 = Empty Array?(array=w457) -> (empty?=w456:bool)
                          n342 = case shown="False" w456 {
                            tunnel: w455 -> [w461 w471]
                            tunnel: w454 -> [w462 _]
                            frame False {
                              n343 = Add(x=w462, y=w461) -> (x+y=w460:dbl)
                              n344 = global read "G_SEN.vi" "vision lane width"() -> (w470:dbl)
                              n345 = Multiply(x=w460, y=0.5) -> (x*y=w458:dbl)
                              n346 = Divide(x=w458, y=w470) -> (x/y=w468:dbl)
                              n347 = local read "Coeff right"() -> (w466:dbl[])
                              n348 = local read "Coeff left"() -> (w469:dbl[])
                              n349 = Decrement(x=w468) -> (x-1=w467:dbl)
                              n350 = Multiply(x=w469, y=w468) -> (x*y=w465:dbl[])
                              n351 = Multiply(x=w467, y=w466) -> (x*y=w464:dbl[])
                              n352 = Subtract(x=w465, y=w464) -> (x-y=w463:dbl[])
                              n353 = global write "G_SEN.vi" "Lane_C_M"(w463) -> ()
                            }
                            frame True {
                              n354 = local read "Coeff right"() -> (w477:dbl[])
                              n355 = Index Array(array=w477, index=0) -> (element=w475:dbl)
                              n356 = Subtract(x=w475, y=w471) -> (x-y=w474:dbl)
                              n357 = Replace Array Subset(array=w477, new element=w474, index=0) -> (w472:dbl[])
                              n358 = global write "G_SEN.vi" "Lane_C_M"(w472) -> ()
                            }
                          }
                        }
                      }
                    }
                    frame 1 {
                      n359 = local read "Rleft"() -> (w481:dbl)
                      n360 = Less Than 0?(x=w481) -> (x < 0?=w479:bool)
                      n361 = case shown="True" w479 {
                        tunnel: w480 -> [_ w502]
                        tunnel: w478 -> [w484 w501]
                        frame False {
                          n362 = local read "Coeff right"() -> (w483:dbl[])
                          n363 = Empty Array?(array=w483) -> (empty?=w482:bool)
                          n364 = case shown="False" w482 {
                            tunnel: w484 -> [w485 w494]
                            frame False {
                              n365 = global read "G_SEN.vi" "vision lane width"() -> (w493:dbl)
                              n366 = Divide(x=w485, y=w493) -> (x/y=w491:dbl)
                              n367 = local read "Coeff right"() -> (w492:dbl[])
                              n368 = local read "Coeff left"() -> (w489:dbl[])
                              n369 = Decrement(x=w491) -> (x-1=w490:dbl)
                              n370 = Multiply(x=w492, y=w491) -> (x*y=w488:dbl[])
                              n371 = Multiply(x=w490, y=w489) -> (x*y=w487:dbl[])
                              n372 = Subtract(x=w488, y=w487) -> (x-y=w486:dbl[])
                              n373 = global write "G_SEN.vi" "Lane_C_M"(w486) -> ()
                            }
                            frame True {
                              n374 = local read "Coeff left"() -> (w500:dbl[])
                              n375 = Index Array(array=w500, index=0) -> (element=w498:dbl)
                              n376 = Add(x=w498, y=w494) -> (x+y=w497:dbl)
                              n377 = Replace Array Subset(array=w500, new element=w497, index=0) -> (w495:dbl[])
                              n378 = global write "G_SEN.vi" "Lane_C_M"(w495) -> ()
                            }
                          }
                        }
                        frame True {
                          n379 = local read "Coeff right"() -> (w504:dbl[])
                          n380 = Empty Array?(array=w504) -> (empty?=w503:bool)
                          n381 = case shown="False" w503 {
                            tunnel: w502 -> [w506 w518]
                            tunnel: w501 -> [w507 _]
                            frame False {
                              n382 = Add(x=w507, y=w506) -> (x+y=w509:dbl)
                              n383 = global read "G_SEN.vi" "vision lane width"() -> (w517:dbl)
                              n384 = Multiply(x=w509, y=0.5) -> (x*y=w505:dbl)
                              n385 = Divide(x=w505, y=w517) -> (x/y=w515:dbl)
                              n386 = local read "Coeff right"() -> (w516:dbl[])
                              n387 = local read "Coeff left"() -> (w513:dbl[])
                              n388 = Decrement(x=w515) -> (x-1=w514:dbl)
                              n389 = Multiply(x=w516, y=w515) -> (x*y=w512:dbl[])
                              n390 = Multiply(x=w514, y=w513) -> (x*y=w511:dbl[])
                              n391 = Subtract(x=w512, y=w511) -> (x-y=w510:dbl[])
                              n392 = global write "G_SEN.vi" "Lane_C_M"(w510) -> ()
                            }
                            frame True {
                              n393 = local read "Coeff left"() -> (w524:dbl[])
                              n394 = Index Array(array=w524, index=0) -> (element=w522:dbl)
                              n395 = Add(x=w522, y=w518) -> (x+y=w521:dbl)
                              n396 = Replace Array Subset(array=w524, new element=w521, index=0) -> (w519:dbl[])
                              n397 = global write "G_SEN.vi" "Lane_C_M"(w519) -> ()
                            }
                          }
                        }
                      }
                    }
                  }
                }
                frame Enabled {
                  n398 = Build Array(w616, w615) -> (w590:dbl[])
                  n399 = global read "G_ALL.vi" "CARSPEC"() -> (w613:T3)
                  n400 = Absolute Value(x=w590) -> (abs(x)=w614:dbl[])
                  n401 = Unbundle By Name(w613) -> ("Overall width"=w612:dbl, "af"=w610:dbl, "Overall width"=w538:dbl)
                  n402 = Array Max & Min(array=w614) -> (max value=w592:dbl, min value=w548:dbl, min index (indices)=w589:i32)  [unwired: 1 out]
                  n403 = global read "G_ALL.vi" "CARSPEC"() -> (w601:T3)
                  n404 = Add(x=w548, y=w612) -> (x+y=w611:dbl)
                  n405 = Index Array(array=w590, index=w589) -> (element=w588:dbl)
                  n406 = Square(x=w610) -> (x^2=w608:dbl)
                  n407 = Not Equal?(x=inf, y=w592) -> (x != y?=w587:bool)
                  n408 = Unbundle By Name(w601) -> ("Overall width"=w532:dbl, "af"=w600:dbl)
                  n409 = Select(t=w592, s=w587, f=w548) -> (s? t:f=w591:dbl)
                  n410 = Square(x=w611) -> (x^2=w609:dbl)
                  n411 = Multiply(x=w538, y=0.5) -> (x*y=w537:dbl)
                  n412 = Add(x=w609, y=w608) -> (x+y=w607:dbl)
                  n413 = Square(x=w591) -> (x^2=w598:dbl)
                  n414 = Square(x=w600) -> (x^2=w599:dbl)
                  n415 = Subtract(x=w598, y=w599) -> (x-y=w549:dbl)
                  n416 = Square Root(x=w607) -> (sqrt(x)=w606:dbl)
                  n417 = global read "G_SEN.vi" "vision lane width"() -> (w604:dbl)
                  n418 = Add(x=w537, y=0.1) -> (x+y=w534:dbl)
                  n419 = Subtract(x=w548, y=w606) -> (x-y=w605:dbl)
                  n420 = Max & Min(x=w549, y=w548) -> (max(x,y)=w547:dbl)  [unwired: 1 out]
                  n421 = global read "G_SEN.vi" "vision lane width"() -> (w596:dbl)
                  n422 = Compound Arithmetic op=ADD(w605, w538, w604) -> (w603:dbl)
                  n423 = Square Root(x=w547) -> (sqrt(x)=w597:dbl)
                  n424 = Multiply(x=0.5, y=w532) -> (x*y=w529:dbl)
                  n425 = Subtract(x=w591, y=w597) -> (x-y=w530:dbl)
                  n426 = Multiply(x=w603, y=0.5) -> (x*y=w535:dbl)
                  n427 = Max & Min(x=w535, y=w534) -> (max(x,y)=w533:dbl)  [unwired: 1 out]
                  n428 = Compound Arithmetic op=ADD(w530, w596) -> (w594:dbl)
                  n429 = Compound Arithmetic op=ADD(0.1 ("value"), w529, w530) -> (w526:dbl)
                  n430 = Multiply(x=w594, y=0.5) -> (x*y=w527:dbl)
                  n431 = Max & Min(x=w526, y=w527) -> (max(x,y)=w525:dbl)  [unwired: 1 out]
                  n432 = case shown="True" w587 {
                    tunnel: w589 -> [w621 w639]
                    tunnel: w588 -> [w620 _]
                    tunnel: w533 -> [w619 w642]
                    tunnel: [w618 w634] -> w586
                    tunnel: w525 -> [w617 w644]
                    frame False {
                      n433 = case shown="1" w621 {
                        tunnel: w620 -> [w626 w633]
                        tunnel: w619 -> [w623 w631]
                        tunnel: [w622 w627] -> w618
                        tunnel: w617 -> [w624 w630]
                        frame 0, Default {
                          n434 = Less Than 0?(x=w626) -> (x < 0?=w625:bool)
                          n435 = Select(t=w624, s=w625, f=w623) -> (s? t:f=w622:dbl)
                        }
                        frame 1 {
                          n436 = Greater Than 0?(x=w633) -> (x > 0?=w632:bool)
                          n437 = global read "G_SEN.vi" "vision lane width"() -> (w629:dbl)
                          n438 = Select(t=w630, s=w632, f=w631) -> (s? t:f=w628:dbl)
                          n439 = Subtract(x=w629, y=w628) -> (x-y=w627:dbl)
                        }
                      }
                    }
                    frame True {
                      n440 = Equal To 0?(x=w639) -> (x = 0?=w638:bool)
                      n441 = global read "G_SEN.vi" "vision lane width"() -> (w645:dbl)
                      n442 = Subtract(x=w645, y=w644) -> (x-y=w643:dbl)
                      n443 = global read "G_SEN.vi" "vision lane width"() -> (w637:dbl)
                      n444 = Add(x=w643, y=w642) -> (x+y=w640:dbl)
                      n445 = Multiply(x=w640, y=0.5) -> (x*y=w636:dbl)
                      n446 = Subtract(x=w637, y=w636) -> (x-y=w635:dbl)
                      n447 = Select(t=w636, s=w638, f=w635) -> (s? t:f=w634:dbl)
                    }
                  }
                  n448 = global read "G_SEN.vi" "vision lane width"() -> (w585:dbl)
                  n449 = local read "Coeff right"() -> (w571:dbl[])
                  n450 = local read "Coeff left"() -> (w558:dbl[])
                  n451 = global read "G_SEN.vi" "vision lane width"() -> (w569:dbl)
                  n452 = global read "G_SEN.vi" "vision lane width"() -> (w560:dbl)
                  n453 = Divide(x=w586, y=w585) -> (x/y=w545:dbl)
                  n454 = local read "poly"() -> (w576:i32)
                  n455 = local read "poly"() -> (w554:i32)
                  n456 = Increment(x=w576) -> (x+1=w575:i32)
                  n457 = Increment(x=w554) -> (x+1=w555:i32)
                  n458 = Index Array(array=w571, index #1=0 ("index")) -> (element #1=w570:dbl, element #2=w551:dbl)  [unwired: 1 in]
                  n459 = Index Array(array=w558, index #1=0 ("index")) -> (element #1=w559:dbl, element #2=w550:dbl)  [unwired: 1 in]
                  n460 = Subtract(x=0.5, y=w545) -> (x-y=w542:dbl)
                  n461 = local read "Coeff right"() -> (w564:dbl[])
                  n462 = Subtract(x=w570, y=w569) -> (x-y=w568:dbl)
                  n463 = Add(x=w559, y=w560) -> (x+y=w561:dbl)
                  n464 = Initialize Array(0.0 ("element"), w575) -> (w574:dbl[])
                  n465 = Initialize Array(0.0 ("element"), w555) -> (w556:dbl[])
                  n466 = local read "Coeff left"() -> (w579:dbl[])
                  n467 = Multiply(x=w542, y="x_gain") -> (x*y=w541:dbl)
                  n468 = Empty Array?(array=w564) -> (empty?=w566:bool)
                  n469 = Empty Array?(array=w579) -> (empty?=w580:bool)
                  n470 = Replace Array Subset(array=w574, new element #1=w568, index #1=0 ("index"), new element #2=w551) -> (w573:dbl[])  [unwired: 1 in]
                  n471 = Replace Array Subset(array=w556, new element #1=w561, index #1=0 ("index"), new element #2=w550) -> (w552:dbl[])  [unwired: 1 in]
                  n472 = Not(x=w566) -> (.not. x?=w565:bool)
                  n473 = Subtract(x=0.5 ("y"), y=w541) -> (x-y=w543:dbl)
                  n474 = Select(t=w573, s=w580, f=w579) -> (s? t:f=w578:dbl[])
                  n475 = Select(t=w564, s=w565, f=w552) -> (s? t:f=w563:dbl[])
                  n476 = Decrement(x=w543) -> (x-1=w584:dbl)
                  n477 = Multiply(x=w578, y=w543) -> (x*y=w582:dbl[])
                  n478 = Multiply(x=w584, y=w563) -> (x*y=w583:dbl[])
                  n479 = Subtract(x=w582, y=w583) -> (x-y=w581:dbl[])
                  n480 = global write "G_SEN.vi" "Lane_C_M"(w581) -> ()
                }
              }
            }
          }
          n481 = Subtract(x=0.5, y=w329) -> (x-y=w331:dbl)
          n482 = Multiply(x=w331, y=2.0) -> (x*y=→"ratio(-1:left1:right)":dbl)
        }
        frame #2 {
          n483 = global read "G_SEN.vi" "Lane_C_M"() -> (w646:dbl[])
          "Lane_C_M" <- w646
          n484 = Index Array(array=w646, index=0) -> (element=w648:dbl)
          n485 = Not A Number/Path/Refnum?(number/path/refnum=w648) -> (NaN/Path/Refnum?=w649:bool)
          n486 = case shown="True" w649 {
            selector: w649 -> [_ w650]
            frame False {
            }
            frame True {
              "NaN/Path/Refnum?" <- w650
            }
          }
        }
      }
    }
    frame #3 {
      n487 = flat-sequence {
        frame #0 {
          n488 = local read "w"() -> (w670:dbl[])
          n489 = Not Equal?(x=w670, y=0.0) -> (x != y?=w663:bool[])
          n490 = global read "G_ALL.vi" "map_track 2"() -> (w654:dbl[][])
          n491 = local read "x"() -> (w668:dbl[])
          n492 = local read "y"() -> (w667:dbl[])
          n493 = Boolean To (0,1)(Boolean=w663) -> (0, 1=w661:i16[])
          n494 = Build Cluster Array(w663, w668, w667) -> (w666:cluster{bool, dbl, dbl}[])
          n495 = To Long Integer(number=w661) -> (32bit integer=w660:i32[])
          n496 = Index Array(array=w654, index (col)=1 ("disabled index (col)")) -> (element=w651:dbl[])  [unwired: 1 in]
          n497 = Add Array Elements(numeric array=w660) -> (sum=w662:i32)
          n498 = Sort 1D Array(array=w666) -> (sorted array=w665:cluster{bool, dbl, dbl}[])
          n499 = Replace Array Subset(array=w654, new element=w651, index (col)=1 ("disabled index (col)")) -> (→"map_track":dbl[][])  [unwired: 1 in]
          n500 = Reverse 1D Array(array=w665) -> (reversed array=w664:cluster{bool, dbl, dbl}[])
          n501 = for {
            N: w662 -> [_]
            tunnel: w664 -> [w674] mode=indexing
            tunnel: [w673] -> w658 mode=indexing
            tunnel: [w672] -> w659 mode=indexing
            tunnel: [w671] -> _
            i -> [w671]
            n502 = Unbundle(w674) -> (w673:dbl, w672:dbl)  [unwired: 1 out]
          }
          n503 = Build Array(w658, w659) -> (w657:dbl[][])
          n504 = Transpose 2D Array(2D array=w657) -> (transposed array=→"lane_pt":dbl[][])
        }
        frame #1 {
          n505 = local read "map_track"() -> (w693:dbl[][])
          n506 = for {
            N: 10 ("Numeric") -> [_]
            shift-right: [w694] -> w687
            shift-left: w693 -> [w702]
            i -> [w701]
            stop <- w697 stop-if-true
            n507 = Array Size(array=w702) -> (size(s)=w714:i32[])
            n508 = Index Array(array=w702, index (col)=1 ("disabled index (col)")) -> (element=w706:dbl[])  [unwired: 1 in]
            n509 = local read "lane_pt"() -> (w719:dbl[][])
            n510 = Index Array(array=w706, index=0) -> (element=w700:dbl)
            n511 = Index Array(array=w714, index=0) -> (element=w712:i32)
            n512 = Subtract(x=w706, y=w700) -> (x-y=w705:dbl[])
            n513 = Index Array(array=w719, index (col) #1=0 ("disabled index (col)")) -> (element #1=w717:dbl[], element #2=w716:dbl[])  [unwired: 3 in]
            n514 = for {
              N: w712 -> [_]
              tunnel: w717 -> [w734]
              tunnel: w716 -> [w729]
              tunnel: "d_safe" -> [w736]
              shift-right: [w720] -> w711
              shift-left: w702 -> [w722]
              i -> [w745]
              n515 = Index Array(array=w722, index (row) #1=w745, index (col) #1=0 ("index"), index (row) #2=w745, index (col) #2=1 ("disabled index (col)")) -> (element #1=w730:dbl, element #2=w724:dbl)
              n516 = Subtract(x=w730, y=w734) -> (x-y=w742:dbl[])
              n517 = Subtract(x=w724, y=w729) -> (x-y=w741:dbl[])
              n518 = Square(x=w742) -> (x^2=w750:dbl[])
              n519 = Square(x=w741) -> (x^2=w749:dbl[])
              n520 = Add(x=w750, y=w749) -> (x+y=w748:dbl[])
              n521 = Square Root(x=w748) -> (sqrt(x)=w747:dbl[])
              n522 = Array Max & Min(array=w747) -> (min value=w738:dbl, min index (indices)=w728:i32)  [unwired: 2 out]
              n523 = Index Array(array=w734, index=w728) -> (element=w733:dbl)
              n524 = Index Array(array=w742, index=w728) -> (element=w740:dbl)
              n525 = Index Array(array=w729, index=w728) -> (element=w727:dbl)
              n526 = Greater?(x=w738, y=w736) -> (0:w746:bool)
              n527 = Index Array(array=w741, index=w728) -> (element=w739:dbl)
              n528 = Divide(x=w740, y=w738) -> (x/y=w737:dbl)
              n529 = Divide(x=w739, y=w738) -> (x/y=w735:dbl)
              n530 = Multiply(x=w737, y=w736) -> (x*y=w732:dbl)
              n531 = Multiply(x=w736, y=w735) -> (x*y=w726:dbl)
              n532 = Add(x=w733, y=w732) -> (x+y=w731:dbl)
              n533 = Add(x=w727, y=w726) -> (x+y=w725:dbl)
              n534 = Subtract(x=w731, y=w730) -> (x-y=w723:dbl)
              n535 = Subtract(x=w725, y=w724) -> (x-y=w721:dbl)
              n536 = case shown="False" w746 {
                tunnel: w723 -> [w752 _]
                tunnel: w722 -> [w766 w767]
                tunnel: w721 -> [w758 _]
                tunnel: [w759 w767] -> w720
                frame False {
                  n537 = In Range and Coerce(upper limit=0.1, x=w752, lower limit=-0.1 ("upper limit")) -> (coerced(x)=w751:dbl)  [unwired: 1 out]
                  n538 = In Range and Coerce(upper limit=0.1, x=w758, lower limit=-0.1 ("upper limit")) -> (coerced(x)=w755:dbl)  [unwired: 1 out]
                  n539 = Index Array(array=w766, index (col) #1=0 ("disabled index (col)")) -> (element #1=w764:dbl[], element #2=w763:dbl[])  [unwired: 3 in]
                  n540 = Add(x=w764, y=w751) -> (x+y=w761:dbl[])
                  n541 = Add(x=w763, y=w755) -> (x+y=w762:dbl[])
                  n542 = Build Array(w761, w762) -> (w760:dbl[][])
                  n543 = Transpose 2D Array(2D array=w760) -> (transposed array=w759:dbl[][])
                }
                frame True {
                }
              }
            }
            n544 = Index Array(array=w711, index (row)=0, index (col)=1 ("disabled index (col)")) -> (element=w699:dbl)
            n545 = Subtract(x=w700, y=w699) -> (x-y=w695:dbl)
            n546 = Add(x=w705, y=w699) -> (x+y=w703:dbl[])
            n547 = Absolute Value(x=w695) -> (abs(x)=w696:dbl)
            n548 = Replace Array Subset(array=w702, new element=w703, index (col)=1 ("disabled index (col)")) -> (w694:dbl[][])  [unwired: 1 in]
            n549 = Less?(x=w696, y=0.05) -> (x < y?=w697:bool)
            "Numeric 2" <- w701
          }
          "map_track 2" <- w687
          n550 = local read "map_track"() -> (w682:dbl[][])
          n551 = Index Array(array=w687, index (row)=0, index (col)=1 ("disabled index (col)")) -> (element=w680:dbl)
          n552 = Index Array(array=w682, index (row)=0, index (col)=1 ("disabled index (col)")) -> (element=w681:dbl)
          n553 = Subtract(x=w680, y=w681) -> (x-y=w679:dbl)
          n554 = Multiply(x=w679, y="y_gain") -> (x*y=w676:dbl)
          n555 = In Range and Coerce(upper limit=0.05, x=w676, lower limit=-0.05 ("upper limit")) -> (coerced(x)=w675:dbl)  [unwired: 1 out]
          n556 = Not A Number/Path/Refnum?(number/path/refnum=w675) -> (NaN/Path/Refnum?=w691:bool)
          n557 = Select(t=0.0, s=w691, f=w675) -> (s? t:f=w689:dbl)
          n558 = local write "y_shift"(w689) -> ()
          n559 = global write "G_SEN.vi" "vision y shift"(w689) -> ()
        }
      }
    }
    frame #4 {
      n560 = local read "w"() -> (→"Waveform Graph":dbl[])
      n561 = local read "w"() -> (w863:dbl[])
      n562 = local read "w"() -> (w843:dbl[])
      n563 = Equal?(x=w863, y=-1.0) -> (x = y?=w861:bool[])
      n564 = Equal?(x=w843, y=1.0) -> (x = y?=w845:bool[])
      n565 = local read "x"() -> (w860:dbl[])
      n566 = local read "y"() -> (w859:dbl[])
      n567 = local read "x"() -> (w846:dbl[])
      n568 = local read "y"() -> (w847:dbl[])
      n569 = Build Cluster Array(w861, w860, w859) -> (w858:cluster{bool, dbl, dbl}[])
      n570 = Build Cluster Array(w845, w846, w847) -> (w848:cluster{bool, dbl, dbl}[])
      n571 = Sort 1D Array(array=w858) -> (sorted array=w857:cluster{bool, dbl, dbl}[])
      n572 = Sort 1D Array(array=w848) -> (sorted array=w849:cluster{bool, dbl, dbl}[])
      n573 = Reverse 1D Array(array=w857) -> (reversed array=w856:cluster{bool, dbl, dbl}[])
      n574 = Reverse 1D Array(array=w849) -> (reversed array=w850:cluster{bool, dbl, dbl}[])
      n575 = for {
        tunnel: w856 -> [w877] mode=indexing
        tunnel: [w875] -> w855 mode=indexing
        tunnel: [w874] -> w836 mode=indexing
        tunnel: [w873] -> w854
        i -> [w873]
        stop <- w876 continue-if-true
        n576 = Unbundle(w877) -> (w876:bool, w875:dbl, w874:dbl)
      }
      n577 = for {
        tunnel: w850 -> [w872] mode=indexing
        tunnel: [w870] -> w851 mode=indexing
        tunnel: [w869] -> w832 mode=indexing
        tunnel: [w868] -> w852
        i -> [w868]
        stop <- w871 continue-if-true
        n578 = Unbundle(w872) -> (w871:bool, w870:dbl, w869:dbl)
      }
      n579 = Array Subset(array=w855, index=0, length=w854) -> (w853:dbl[])
      n580 = Array Subset(array=w836, index=0, length=w854) -> (w831:dbl[])
      n581 = Array Subset(array=w851, index=0, length=w852) -> (w842:dbl[])
      n582 = Array Subset(array=w832, index=0, length=w852) -> (w827:dbl[])
      n583 = call "Convert to Dynamic Data4"("Array"=w853) -> ("Dynamic Data Type"=w816:dynamicdata)  [unwired: 3 in]
      n584 = Array Max & Min(array=w831) -> (max value=w838:dbl, min value=w837:dbl)  [unwired: 2 out]
      n585 = call "Convert to Dynamic Data3"("Array"=w831) -> ("Dynamic Data Type"=w828:dynamicdata)  [unwired: 3 in]
      n586 = call "Convert to Dynamic Data6"("Array"=w842) -> ("Dynamic Data Type"=w814:dynamicdata)  [unwired: 3 in]
      n587 = Array Max & Min(array=w827) -> (max value=w834:dbl, min value=w835:dbl)  [unwired: 2 out]
      n588 = call "Convert to Dynamic Data8"("Array"=w827) -> ("Dynamic Data Type"=w826:dynamicdata)  [unwired: 3 in]
      n589 = Increment(x=w838) -> (x+1=w799:dbl)
      n590 = Decrement(x=w837) -> (x-1=w794:dbl)
      n591 = Increment(x=w834) -> (x+1=w798:dbl)
      n592 = Decrement(x=w835) -> (x-1=w793:dbl)
      n593 = local read "map_track"() -> (w774:dbl[][])
      n594 = Add(x=w799, y=w798) -> (x+y=w797:dbl)
      n595 = Add(x=w794, y=w793) -> (x+y=w791:dbl)
      n596 = call-poly <vilib>:"Ramp Pattern.vi"("start"=w794, "end"=w799, "delta"=0.01) -> ("Ramp Pattern"=w803:dbl[])  [unwired: 6 in, 2 out]
      n597 = call-poly <vilib>:"Ramp Pattern.vi"("start"=w793, "end"=w798, "delta"=0.01) -> ("Ramp Pattern"=w802:dbl[])  [unwired: 6 in, 2 out]
      n598 = local read "Coeff right"() -> (w801:dbl[])
      n599 = local read "Coeff stop"() -> (w841:dbl[])
      n600 = local read "Coeff left"() -> (w866:dbl[])
      n601 = Index Array(array=w774, index (col) #1=0 ("disabled index (col)")) -> (element #1=w778:dbl[], element #2=w780:dbl[])  [unwired: 3 in]
      n602 = Multiply(x=w797, y=0.5) -> (x*y=w795:dbl)
      n603 = Multiply(x=w791, y=0.5) -> (x*y=w790:dbl)
      n604 = local read "map_track 2"() -> (w773:dbl[][])
      n605 = call-poly <vilib>:"Polynomial Evaluation.vi"("P(x)"=w866, "A"=w803) -> ("P(A)"=w809:dbl[])  [unwired: 1 out]
      n606 = call-poly <vilib>:"Polynomial Evaluation.vi"("P(x)"=w801, "A"=w802) -> ("P(A)"=w804:dbl[])  [unwired: 1 out]
      n607 = call "Convert to Dynamic Data7"("Array"=w803) -> ("Dynamic Data Type"=w813:dynamicdata)  [unwired: 3 in]
      n608 = call "Convert to Dynamic Data11"("Array"=w802) -> ("Dynamic Data Type"=w812:dynamicdata)  [unwired: 3 in]
      n609 = local read "y_end"() -> (w840:dbl[])
      n610 = call-poly <vilib>:"Ramp Pattern.vi"("start"=w790, "end"=w795, "delta"=0.01) -> ("Ramp Pattern"=w786:dbl[])  [unwired: 6 in, 2 out]
      n611 = global read "G_SEN.vi" "Lane_C_M"() -> (w789:dbl[])
      n612 = Add(x=w778, y="x_shift") -> (x+y=w777:dbl[])
      n613 = Add(x=w780, y="y_shift") -> (x+y=w779:dbl[])
      n614 = call-poly <vilib>:"Polynomial Evaluation.vi"("P(x)"=w841, "A"=w840) -> ("P(A)"=w810:dbl[])  [unwired: 1 out]
      n615 = Build Array(w809, w803) -> (w808:dbl[][])
      n616 = Build Array(w804, w802) -> (w805:dbl[][])
      n617 = call "Convert to Dynamic Data2"("Array"=w809) -> ("Dynamic Data Type"=w817:dynamicdata)  [unwired: 3 in]
      n618 = call "Convert to Dynamic Data5"("Array"=w804) -> ("Dynamic Data Type"=w815:dynamicdata)  [unwired: 3 in]
      n619 = Index Array(array=w773, index (col) #1=0 ("disabled index (col)")) -> (element #1=w771:dbl[], element #2=w769:dbl[])  [unwired: 3 in]
      n620 = local read "y"() -> (w865:dbl[])
      n621 = local read "y_end"() -> (w811:dbl[])
      n622 = call-poly <vilib>:"Polynomial Evaluation.vi"("P(x)"=w789, "A"=w786) -> ("P(A)"=w788:dbl[])  [unwired: 1 out]
      n623 = Transpose 2D Array(2D array=w808) -> (transposed array=w807:dbl[][])
      n624 = Transpose 2D Array(2D array=w805) -> (transposed array=w806:dbl[][])
      n625 = call "Convert to Dynamic Data14"("Array"=w786) -> ("Dynamic Data Type"=w785:dynamicdata)  [unwired: 3 in]
      n626 = call "Convert to Dynamic Data15"("Array"=w777) -> ("Dynamic Data Type"=w783:dynamicdata)  [unwired: 3 in]
      n627 = call "Convert to Dynamic Data16"("Array"=w779) -> ("Dynamic Data Type"=w782:dynamicdata)  [unwired: 3 in]
      n628 = call "Convert to Dynamic Data17"("Array"=w771) -> ("Dynamic Data Type"=w770:dynamicdata)  [unwired: 3 in]
      n629 = call "Convert to Dynamic Data18"("Array"=w769) -> ("Dynamic Data Type"=w768:dynamicdata)  [unwired: 3 in]
      n630 = call "Convert to Dynamic Data"("Array"=w810) -> ("Dynamic Data Type"=w822:dynamicdata)  [unwired: 3 in]
      n631 = call "Convert to Dynamic Data10"("Array"=w865) -> ("Dynamic Data Type"=w824:dynamicdata)  [unwired: 3 in]
      n632 = local read "x"() -> (w864:dbl[])
      n633 = global write "G_SEN.vi" "Lane_L_V"(w807) -> ()
      n634 = global write "G_SEN.vi" "Lane_R_V"(w806) -> ()
      n635 = Merge Signals(w813, w828, w812, w826, w824, w822, w785, w782, w768) -> (w829:dynamicdata)
      n636 = call "Convert to Dynamic Data12"("Array"=w811) -> ("Dynamic Data Type"=w823:dynamicdata)  [unwired: 3 in]
      n637 = call "Convert to Dynamic Data13"("Array"=w788) -> ("Dynamic Data Type"=w787:dynamicdata)  [unwired: 3 in]
      n638 = call "Convert to Dynamic Data9"("Array"=w864) -> ("Dynamic Data Type"=w825:dynamicdata)  [unwired: 3 in]
      n639 = Merge Signals(w817, w816, w815, w814, w825, w823, w787, w783, w770) -> (w830:dynamicdata)
      n640 = call "Build XY Graph"("Y Input"=w829, "X Input"=w830) -> ("XY Graph"=→"XY Graph 4":cluster{"X":dbl[], "Y":dbl[]}[])  [unwired: 8 in, 1 out]
    }
  }
